vi "BuildTestName.vi"(4 "QualisysDataType":enum16{"6DOF", "3DTracking", "6DOF + 3D"}(ring), 5 "entrée d'erreur":errorcluster, 6 "WhichPath?":T1=enum."Meas", 7 "NextTestNum":u32, 8 "NomProjet":string) -> (0 "sortie d'erreur":errorcluster, 1 "cheminProchainFichier":path, 2 "NomProchainFichier":string, 3 "NomProjetOut":string)   [LabVIEW 2017]
doc: "Ce VI renvoie le nombre de fichier de mesures présents dans le repertoire du projet en cours"
uses:
  DefDeType/WhichPath.ctl
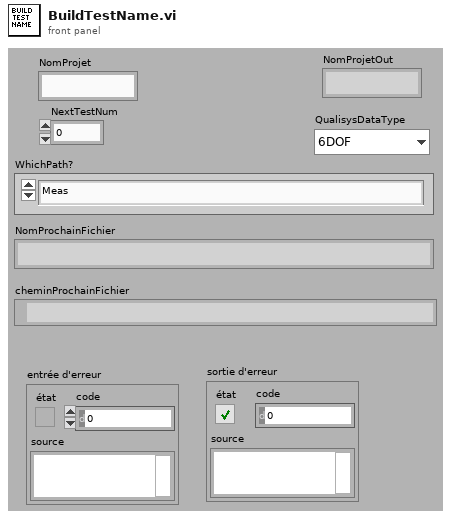
[diagram p1: front panel]
types:
  T1 = typedef "WhichPath.ctl" = enum16{"DossierProjet", "Config", "Meas", "MeasPCI", "MeasCRIO1", "MeasCRIO2", "MeasQualisys", "MeasHBM", "MeasTDMS", "Fig", "Res"}
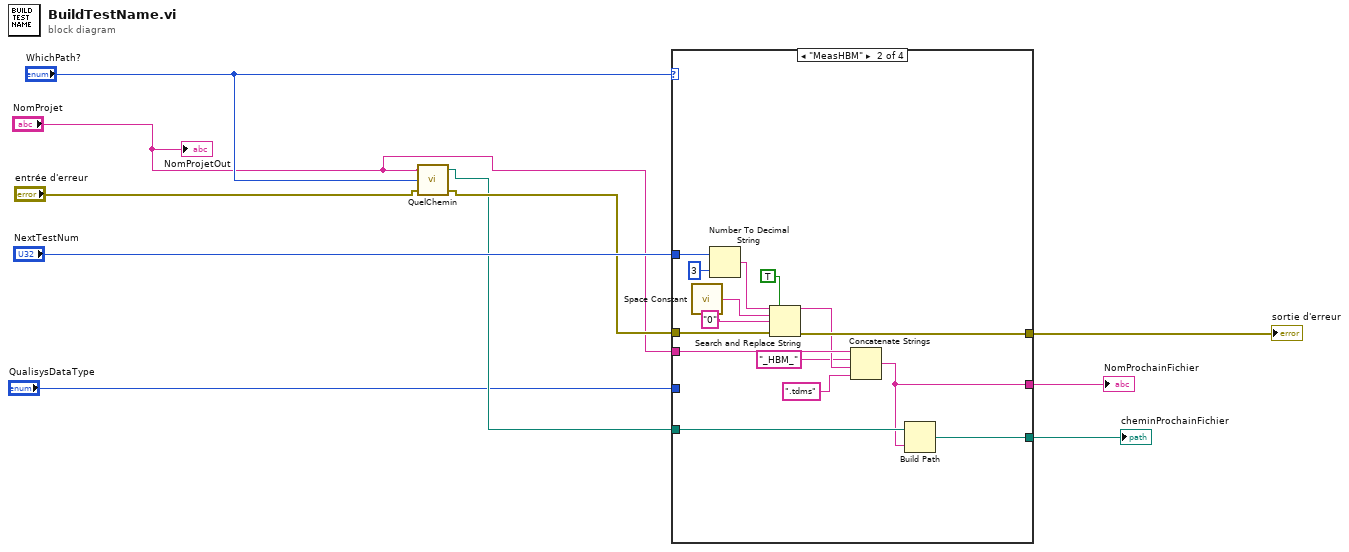
[diagram p0: block diagram]
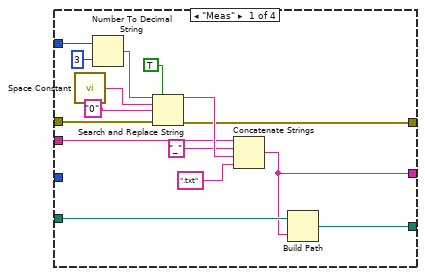
[diagram p2: hidden frame]
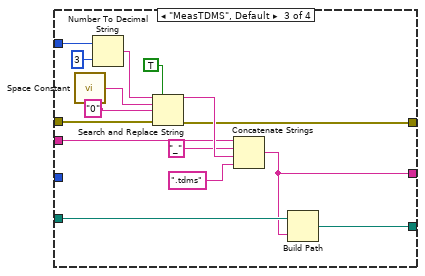
[diagram p3: hidden frame]
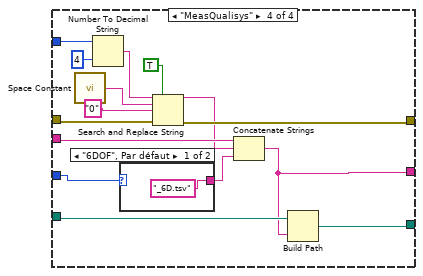
[diagram p4: hidden frame]
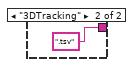
[diagram p5: hidden frame]
diagram:
  n1 = call "QuelChemin.vi"("Entrée d'erreur"="entrée d'erreur", "WhichPath?"="WhichPath?", "NomProjet"="NomProjet") -> ("Sortie d'erreur"=w5:errorcluster, "SurDisqueLocal"=w3:path)  [unwired: 1 out]
  n2 = case shown="\"MeasHBM\"" "WhichPath?" {
    tunnel: w3 -> [w18 w35 w48 w59]
    tunnel: [w17 w34 w47 w58] -> w10
    tunnel: [w15 w32 w45 w57] -> w9
    tunnel: "NextTestNum" -> [w14 w31 w44 w64]
    tunnel: [w13 w30 w43 w62] -> w7
    tunnel: "NomProjet" -> [w12 w29 w42 w61]
    tunnel: w5 -> [w11 w28 w41 w63]
    tunnel: "QualisysDataType" -> [_ _ _ w56]
    frame "Meas" {
      n3 = call <vilib>:"Space Constant.vi"() -> ("String"=w23:string)
      n4 = Number To Decimal String(number=w14, width (-)=i16 3 ("largeur (-)")) -> (decimal integer string=w24:string)
      n5 = Search and Replace String(replace all?=TRUE ("tout remplacer ? (F)"), input string=w24, search string=w23, replace string="0" ("chaîne de remplacement (\"\")"), error in=w11) -> (result string=w21:string, error out=w13:errorcluster)  [unwired: 3 in, 2 out]
      n6 = Concatenate Strings(w12, "_" ("chaîne"), w21, ".txt" ("chaîne")) -> (w15:string)
      n7 = Build Path(base path=w18, name or relative path=w15) -> (appended path=w17:path)
    }
    frame "MeasHBM" {
      n8 = call <vilib>:"Space Constant.vi"() -> ("String"=w38:string)
      n9 = Number To Decimal String(number=w31, width (-)=i16 3 ("largeur (-)")) -> (decimal integer string=w39:string)
      n10 = Search and Replace String(replace all?=TRUE ("tout remplacer ? (F)"), input string=w39, search string=w38, replace string="0" ("chaîne de remplacement (\"\")"), error in=w28) -> (result string=w27:string, error out=w30:errorcluster)  [unwired: 3 in, 2 out]
      n11 = Concatenate Strings(w29, "_HBM_" ("chaîne"), w27, ".tdms" ("chaîne")) -> (w32:string)
      n12 = Build Path(base path=w35, name or relative path=w32) -> (appended path=w34:path)
    }
    frame "MeasTDMS", Default {
      n13 = call <vilib>:"Space Constant.vi"() -> ("String"=w53:string)
      n14 = Number To Decimal String(number=w44, width (-)=i16 3 ("largeur (-)")) -> (decimal integer string=w54:string)
      n15 = Search and Replace String(replace all?=TRUE ("tout remplacer ? (F)"), input string=w54, search string=w53, replace string="0" ("chaîne de remplacement (\"\")"), error in=w41) -> (result string=w51:string, error out=w43:errorcluster)  [unwired: 3 in, 2 out]
      n16 = Concatenate Strings(w42, "_" ("chaîne"), w51, ".tdms" ("chaîne")) -> (w45:string)
      n17 = Build Path(base path=w48, name or relative path=w45) -> (appended path=w47:path)
    }
    frame "MeasQualisys" {
      n18 = call <vilib>:"Space Constant.vi"() -> ("String"=w68:string)
      n19 = Number To Decimal String(number=w64, width (-)=i16 4 ("largeur (-)")) -> (decimal integer string=w69:string)
      n20 = case shown="\"6DOF\", Par défaut" w56 {
        tunnel: ["_6D.tsv" ("chaîne") ".tsv" ("chaîne")] -> w65
        frame "6DOF", Default {
        }
        frame "3DTracking" {
        }
      }
      n21 = Search and Replace String(replace all?=TRUE ("tout remplacer ? (F)"), input string=w69, search string=w68, replace string="0" ("chaîne de remplacement (\"\")"), error in=w63) -> (result string=w60:string, error out=w62:errorcluster)  [unwired: 3 in, 2 out]
      n22 = Concatenate Strings(w61, w60, w65) -> (w57:string)
      n23 = Build Path(base path=w59, name or relative path=w57) -> (appended path=w58:path)
    }
  }
  "cheminProchainFichier" <- w10
  "NomProchainFichier" <- w9
  "sortie d'erreur" <- w7
  "NomProjetOut" <- "NomProjet"
